vi "Globals.vi"() -> ()   [LabVIEW 2017, in "DFD FXP Simulation with State.xnode"]
uses:
  <vilib>/addons/Digital Filter Design/FXPSim.llb/SimXnodewithState/DFD FXP Simulation with State.xnode
  <vilib>/XNodeSupport/XNodeRect32.ctl
  <vilib>/XNodeSupport/XNodeInt.ctl
  <vilib>/XNodeSupport/NI_XNodeSupport.lvlib
panel:
  in  "TERM State out Bound":T1={"Left"=16, "Top"=16, "Right"=24, "Bottom"=32}
  in  "TERM State in Bound":T1={"Left"=8, "Top"=16, "Right"=16, "Bottom"=32}
  in  "TERM State in NAME":string="state in"
  in  "TERM State in ID":string="state in"
  in  "TERM State out NAME":string="state out"
  in  "TERM State out ID":string="state out"
  in  "TERM Statistics out Bound":T1={"Left"=24, "Top"=16, "Right"=32, "Bottom"=24}
  in  "TERM Error out Bound":T1={"Left"=24, "Top"=24, "Right"=32, "Bottom"=32}
  in  "TERM integer out Bound":T1={"Left"=24, "Top"=8, "Right"=32, "Bottom"=16}
  in  "TERM DBL out Bound":T1={"Left"=24, "Top"=0, "Right"=32, "Bottom"=8}
  in  "TERM Input range NAME":string="input range"
  in  "TERM Input range ID":string="input range"
  in  "TERM Integer out NAME":string="integer signal out"
  in  "TERM Integer out ID":string="integer signal out"
  in  "TERM Double out NAME":string="DBL signal out"
  in  "TERM Double out ID":string="DBL signal out"
  in  "TERM Input range Bound":T1={"Left"=16, "Top"=0, "Right"=24, "Bottom"=16}
  in  "TERM Error in Bound":T1={"Left"=0, "Top"=24, "Right"=8, "Bottom"=32}
  in  "TERM Statistics in Bound":T1={"Left"=0, "Top"=16, "Right"=8, "Bottom"=24}
  in  "TERM Filter Bound":T1={"Left"=0, "Top"=8, "Right"=8, "Bottom"=16}
  in  "TERM Signal in Bound":T1={"Left"=0, "Top"=0, "Right"=8, "Bottom"=8}
  in  "TERM Staticstics out NAME":string="filtering staticstics report"
  in  "TERM Statistics out ID":string="filtering statistics report"
  in  "TERM Error out NAME":string="error out"
  in  "TERM Error out ID":string="error out"
  in  "TERM Staticstics in NAME":string="filtering statistics in"
  in  "TERM Statistics in ID":string="filtering statistics in"
  in  "TERM Error in NAME":string="error in (no error)"
  in  "TERM Filter NAME":string="filter in"
  in  "TERM Signal in NAME":string="signal in"
  in  "TERM Error in ID":string="error in (no error)"
  in  "TERM Filter ID":string="filter in"
  in  "TERM Signal in ID":string="signal in"
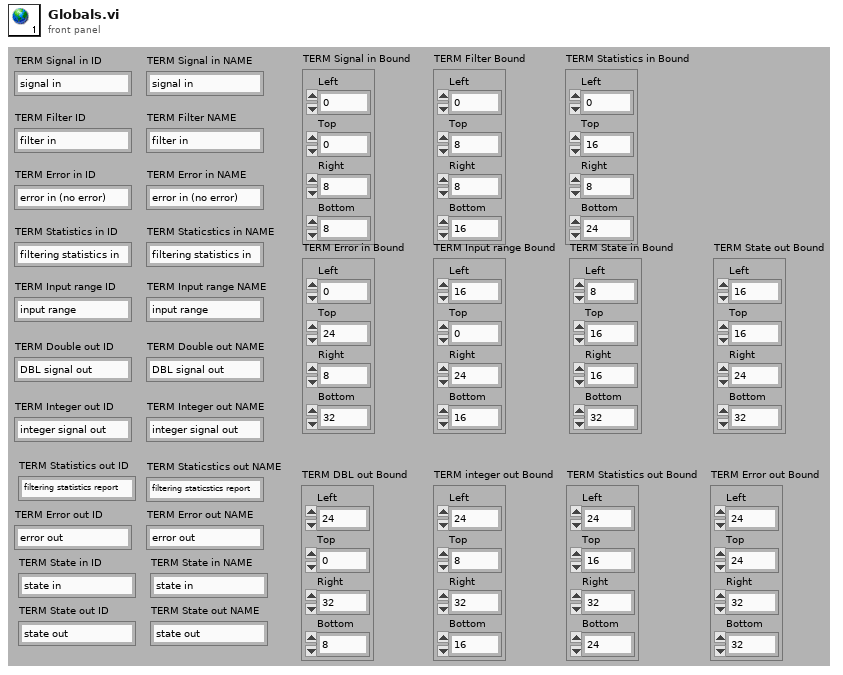
[diagram p1: front panel]
types:
  T1 = typedef "NI_XNodeSupport.lvlib/XNodeRect32.ctl" = cluster{"Left":T2, "Top":T2, "Right":T2, "Bottom":T2}
  T2 = typedef "NI_XNodeSupport.lvlib/XNodeInt.ctl" = i32
diagram:
